vi "XL320_Play Motion.vi"(8 "Compiled motion":T1, 11 "Com Port":refnum<visa-resource-name>="COM1" caption="Com Port (Default COM1)") -> (0 "error out":errorcluster)   [LabVIEW 2015]
doc: "Plays back a motion sequence for the Dynamixel motors. Use the global variable <B>Stop Playback</B> to stop the playback."
uses:
  <instrlib>/Dynamixel XL320/Examples/Record And Playback Motion/Type Defs/XL320_Compiled Motion.ctl
  <vilib>/Platform/TimedLoop/XDataNode/timing_clust.ctl
  <vilib>/Platform/TimedLoop/XDataNode/nitl_modes.ctl
  <vilib>/Platform/TimedLoop/XDataNode/wakeup.ctl
  <vilib>/Platform/TimedLoop/XDataNode/XDataNode.xnode
  <vilib>/Platform/TimedLoop/XDataNode/XDNodeRunTimeDep.lvlib
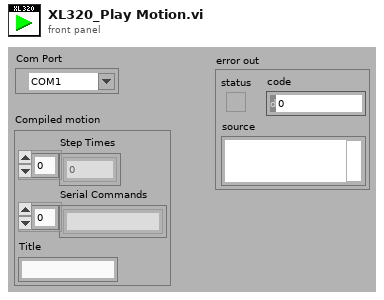
[diagram p1: front panel]
types:
  T1 = typedef "XL320_Compiled Motion.ctl" = cluster{"Step Times":dbl[], "Serial Commands":string[], "Title":string}
  T2 = typedef "XDNodeRunTimeDep.lvlib/timing_clust.ctl" = cluster{"Expected End [f-1]":u64, "Actual End [f-1]":u64, "Finished Late? [f-1]":bool, "Expected End [i-1]":u64, "Actual End [i-1]":u64, "Finished Late? [i-1]":bool, "Expected Start [i]":u64, "Actual Start [i]":u64, "Expected Start [f]":u64, "Actual Start [f]":u64, "Source Name":string, "Structure Name":string, "Period":i64, "Deadline":i64, "Offset":i64, "Start":i64, "Priority":i32, "Timeout":i32, "Mode":T3, "Wakeup Reason":T4, "Error":errorcluster, "Source Type":string, "Secondary Source Type":string, "Global End Time":u64, "Global Start Time":u64, "Frame Duration":u64, "Iteration Duration":u64, "Assigned CPU":i32, "I/O Scan Engine Mode":u32}
  T3 = typedef "XDNodeRunTimeDep.lvlib/nitl_modes.ctl" = enum32{"No Change", "Process missed periods, maintain original phase", "Discard missed periods, maintain original phase", "Process missed periods, ignore original phase", "Discard missed periods, ignore original phase"}
  T4 = typedef "XDNodeRunTimeDep.lvlib/wakeup.ctl" = enum32{"Normal", "Aborted", "Asynchronous wakeup", "Timing source error", "Timed loop error", "Timeout"}
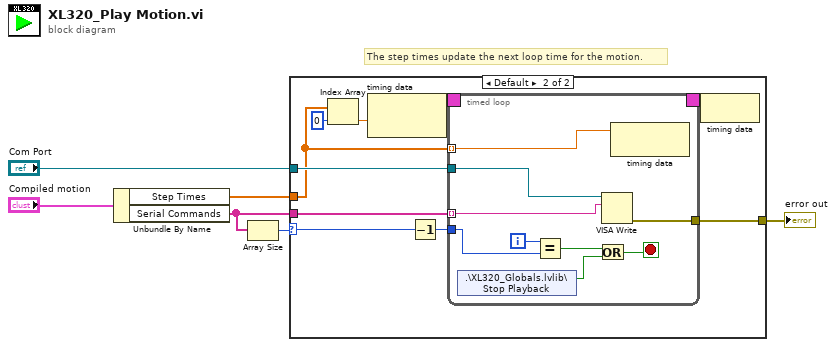
[diagram p0: block diagram]
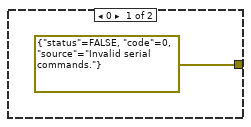
[diagram p2: hidden frame]
diagram:
  # "The step times update the next loop time for the motion."
  n1 = Unbundle By Name("Compiled motion") -> ("Step Times"=w4:dbl[], "Serial Commands"=w5:string[])
  n2 = Array Size(array=w5) -> (size(s)=w2:i32)
  n3 = case shown="Default" w2 {
    selector: w2 -> [_ w8]
    tunnel: "Com Port" -> [_ w13]
    tunnel: w5 -> [_ w12]
    tunnel: w4 -> [_ w11]
    tunnel: [errorcluster {"status"=FALSE, "code"=0, "source"="Invalid serial commands."} ("error out") w9] -> w3
    frame 0 {
    }
    frame Default {
      n4 = Index Array(array=w11, index=0) -> (element=w14:dbl)
      n5 = node-c288(w14) -> (w17:T2)
      n6 = Decrement(x=w8) -> (x-1=w10:i32)
      n7 = timed-loop {
        timing: w17 -> [_]
        timing-out: [_] -> w16
        tunnel: w10 -> [w26]
        tunnel: w11 -> [w23] mode=indexing
        tunnel: w13 -> [w22]
        tunnel: w12 -> [w21] mode=indexing
        tunnel: [w18] -> w9
        i -> [w25]
        stop <- w19 stop-if-true
        n8 = shared-variable ".\\XL320_Globals.lvlib\\Stop Playback"() -> (w20:bool)  [unwired: 1 in, 1 out]
        n9 = Equal?(x=w25, y=w26) -> (x = y?=w24:bool)
        n10 = Or(x=w24, y=w20) -> (x .or. y?=w19:bool)
        n11 = VISA Write(VISA resource name=w22, write buffer=w21) -> (error out=w18:errorcluster)  [unwired: 1 in, 2 out]
        n12 = node-c288(w23) -> ()  [unwired: 1 out]
      }
      n13 = node-c288(w16) -> ()
    }
  }
  "error out" <- w3
